vi "Value Strings.vi"(8 "error in (no error)":errorcluster, 11 "Group in":refnum<class "Group.lvclass">) -> (0 "error out":errorcluster, 2 "Value Strings":string[](array[string]), 3 "Group out":refnum<class "Group.lvclass">)   [LabVIEW 2020, in "Vecto.lvlib" / "Group.lvclass"]
uses:
  Group.lvclass
  Group.lvclass/Group.ctl
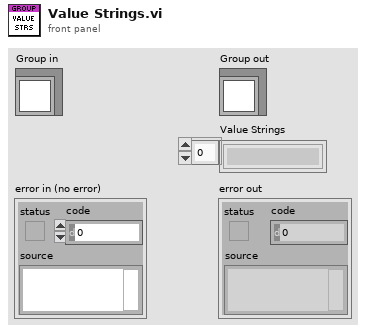
[diagram p1: front panel]
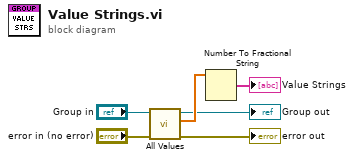
[diagram p0: block diagram]
diagram:
  n1 = call "All Values.vi"("error in (no error)"="error in (no error)", "Group in"="Group in") -> ("error out"=→"error out":errorcluster, "Scaled"=w4:dbl[], "Group out"=→"Group out":refnum<class "Group.lvclass">)  [unwired: 5 in, 2 out]
  n2 = Number To Fractional String(number=w4) -> (F-format string=→"Value Strings":string[])  [unwired: 3 in]
